vi "SineWave.vi"() -> ()   [LabVIEW 2020]
panel:
  in  "stop":bool
  out "Waveform Graph 2":dynamicdata(graph)
  in  "Ok":bool
  out "Waveform Graph":dynamicdata(graph)
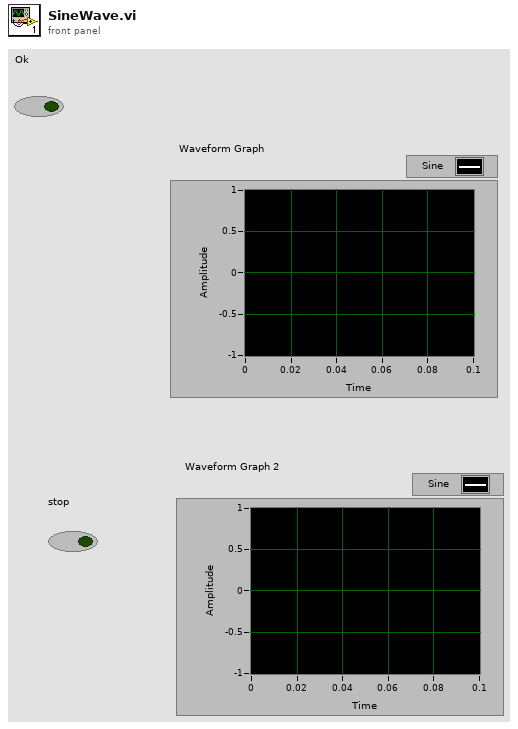
[diagram p1: front panel]
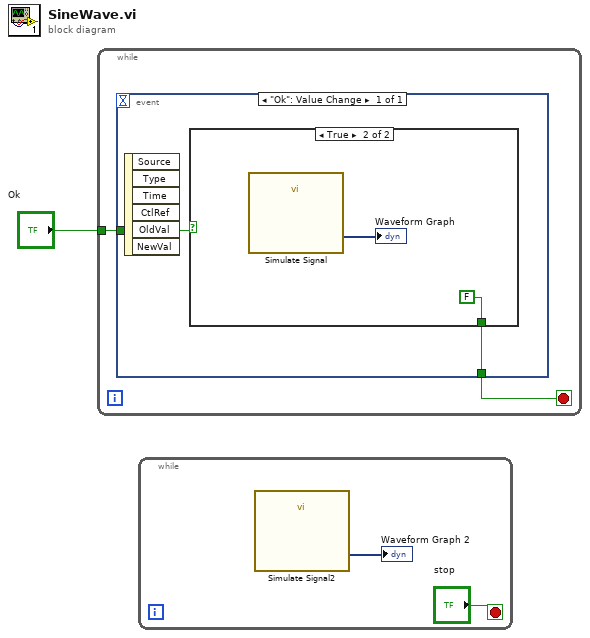
[diagram p0: block diagram]
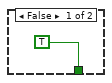
[diagram p2: hidden frame]
diagram:
  n1 = while {
    tunnel: "Ok" -> [w3]
    stop <- w2 stop-if-true
    n2 = event shown="[0] \"Ok\": Value Change" {
      selector: _ -> [_]
      dyn-events: _ -> [_]
      timeout: _ -> [_]
      tunnel: w3 -> [w5]
      tunnel: [w4] -> w2
      event "Ok": Value Change {
        n3 = event-data() -> ()  [unwired: 1 in, 6 out]
        n4 = case shown="True" w5 {
          tunnel: [TRUE FALSE] -> w4
          frame False {
          }
          frame True {
            n5 = call "Simulate Signal"() -> ("Sine"=→"Waveform Graph":dynamicdata)  [unwired: 14 in, 1 out]
          }
        }
      }
    }
  }
  n6 = while {
    stop <- "stop" stop-if-true
    n7 = call "Simulate Signal2"() -> ("Sine"=→"Waveform Graph 2":dynamicdata)  [unwired: 14 in, 1 out]
  }
